vi "AutoCargoShip.vi"(6 "DestinationName":string, 10 "FeederStation":dbl[](array[numeric]), 11 "Coordinates":dbl[](array[numeric])) -> ()   [LabVIEW 2018]
uses:
  Globals.vi
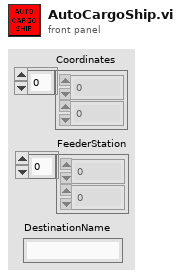
[diagram p1: front panel]
types:
  T1 = enum16{"DriveToHatch", "VisionAlign", "PlaceHatch", "DriveToFeeder"}
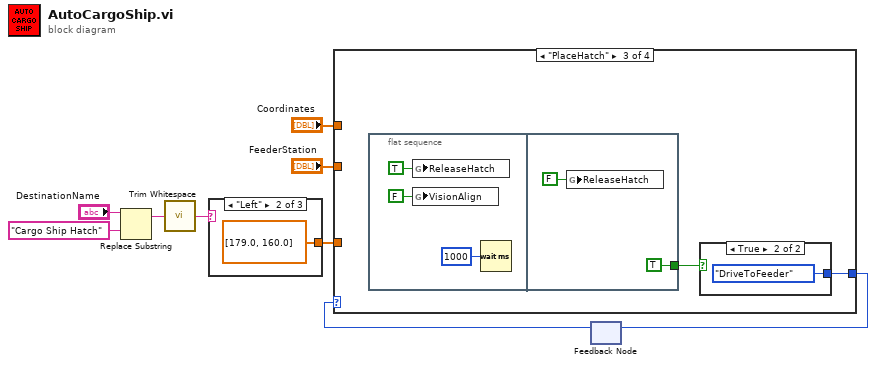
[diagram p0: block diagram]
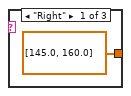
[diagram p2: hidden frame]
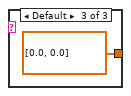
[diagram p3: hidden frame]
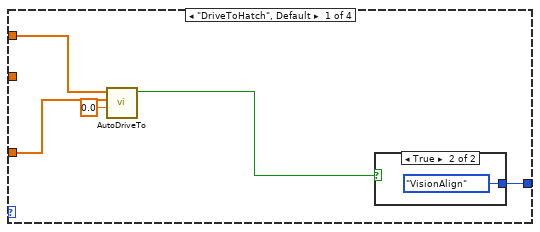
[diagram p4: hidden frame]
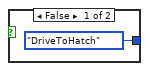
[diagram p5: hidden frame]
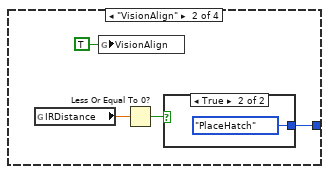
[diagram p6: hidden frame]
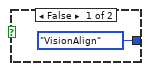
[diagram p7: hidden frame]
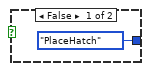
[diagram p8: hidden frame]
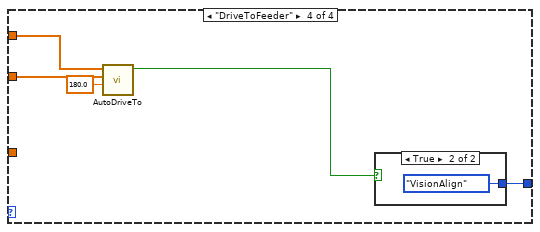
[diagram p9: hidden frame]
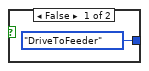
[diagram p10: hidden frame]
diagram:
  n1 = Replace Substring(4:"Cargo Ship Hatch" ("substring (\"\")"), 5:"DestinationName") -> (1:w5:string)  [unwired: 2 in, 1 out]
  n2 = call <vilib>:"Trim Whitespace.vi"("string"=w5) -> ("trimmed string"=w4:string)  [unwired: 1 in]
  n3 = case shown="\"Left\"" w4 {
    tunnel: [dbl[] [145.0, 160.0] dbl[] [179.0, 160.0] dbl[] [0.0, 0.0]] -> w3
    frame "Right" {
    }
    frame "Left" {
    }
    frame Default {
    }
  }
  n4 = feedback #1() -> (w1:T1)  [unwired: 1 in]
  n5 = case shown="\"PlaceHatch\"" w1 {
    tunnel: "Coordinates" -> [w17 _ _ w39]
    tunnel: "FeederStation" -> [_ _ _ w38]
    tunnel: w3 -> [w15 _ _ _]
    tunnel: [w13 w20 w26 w35] -> w2
    frame "DriveToHatch", Default {
      n6 = call "AutoDriveTo.vi"("EndAngle"=0.0, "EndCoordinates"=w15, "Coordinates"=w17) -> ("ThereYet?"=w16:bool)  [unwired: 8 in]
      n7 = case shown="True" w16 {
        tunnel: [T1."DriveToHatch" T1."VisionAlign"] -> w13
        frame False {
        }
        frame True {
        }
      }
    }
    frame "VisionAlign" {
      n8 = global read "Globals.vi" "IRDistance"() -> (w22:dbl)
      n9 = global write "Globals.vi" "VisionAlign"(TRUE ("VisionAlign")) -> ()
      n10 = Less Or Equal To 0?(x=w22) -> (x <= 0?=w21:bool)
      n11 = case shown="True" w21 {
        tunnel: [T1."VisionAlign" T1."PlaceHatch"] -> w20
        frame False {
        }
        frame True {
        }
      }
    }
    frame "PlaceHatch" {
      n12 = flat-sequence {
        tunnel: [TRUE ("VisionAlign")] -> w27
        frame #0 {
          n13 = global write "Globals.vi" "ReleaseHatch"(TRUE ("ReleaseHatch")) -> ()
          n14 = global write "Globals.vi" "VisionAlign"(FALSE ("VisionAlign")) -> ()
          n15 = Wait (ms)(milliseconds to wait=u32 1000) -> ()  [unwired: 1 out]
        }
        frame #1 {
          n16 = global write "Globals.vi" "ReleaseHatch"(FALSE ("ReleaseHatch")) -> ()
        }
      }
      n17 = case shown="True" w27 {
        tunnel: [T1."PlaceHatch" T1."DriveToFeeder"] -> w26
        frame False {
        }
        frame True {
        }
      }
    }
    frame "DriveToFeeder" {
      n18 = call "AutoDriveTo.vi"("EndAngle"=180.0, "EndCoordinates"=w38, "Coordinates"=w39) -> ("ThereYet?"=w36:bool)  [unwired: 8 in]
      n19 = case shown="True" w36 {
        tunnel: [T1."DriveToFeeder" T1."VisionAlign"] -> w35
        frame False {
        }
        frame True {
        }
      }
    }
  }
  n20 = feedback-in #1(w2) -> ()
